vi "subTiE_Deinitialize.vi"(11 "Ref":T1 caption="Ref (can be hidden)") -> ()   [LabVIEW 2015]
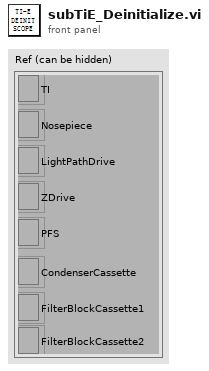
[diagram p1: front panel]
types:
  T1 = cluster{"TI":refnum<k7>, "Nosepiece":refnum<k7>, "LightPathDrive":refnum<k7>, "ZDrive":refnum<k7>, "PFS":refnum<k7>, "CondenserCassette":refnum<k7>, "FilterBlockCassette1":refnum<k7>, "FilterBlockCassette2":refnum<k7>}
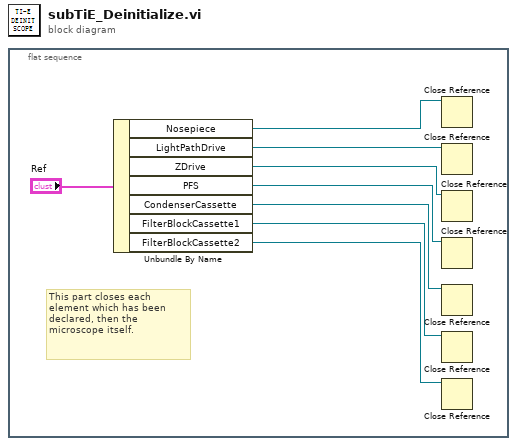
[diagram p0: block diagram]
diagram:
  n1 = flat-sequence {
    frame #0 {
      # "This part closes each element which has been declared, then the microscope itself."
      n2 = Unbundle By Name("Ref") -> ("Nosepiece"=w8:refnum<k7>, "LightPathDrive"=w7:refnum<k7>, "ZDrive"=w6:refnum<k7>, "PFS"=w5:refnum<k7>, "CondenserCassette"=w4:refnum<k7>, "FilterBlockCassette1"=w3:refnum<k7>, "FilterBlockCassette2"=w2:refnum<k7>)
      n3 = Close Reference(reference=w8) -> ()  [unwired: 1 in, 1 out]
      n4 = Close Reference(reference=w7) -> ()  [unwired: 1 in, 1 out]
      n5 = Close Reference(reference=w6) -> ()  [unwired: 1 in, 1 out]
      n6 = Close Reference(reference=w5) -> ()  [unwired: 1 in, 1 out]
      n7 = Close Reference(reference=w4) -> ()  [unwired: 1 in, 1 out]
      n8 = Close Reference(reference=w3) -> ()  [unwired: 1 in, 1 out]
      n9 = Close Reference(reference=w2) -> ()  [unwired: 1 in, 1 out]
    }
  }
